vi "Cascade Logic.vi"(8 "Bank1 Status":T2, 9 "Bank1 Data":T4, 10 "Bank0 Status":T2, 11 "Bank0 Data":T4) -> (0 "Output Valid":bool, 3 "Output Data":T3, 4 "Cascaded Bank Status":T1)   [LabVIEW 2012]
doc: "This VI implements cascade logic to combine two DRAM Banks to act as a single FIFO.\nIt has the higher efficiency in throughput than Ping-Ponging between banks."
uses:
  <userlib>/FPGA Library/Code Development/DRAM/2 Bank DRAM/Data Type (256).ctl
  <userlib>/FPGA Library/Code Development/DRAM/2 Bank DRAM/Controls/Individual Bank Status.ctl
  <userlib>/FPGA Library/Code Development/DRAM/2 Bank DRAM/Controls/Cascaded Bank Status.ctl
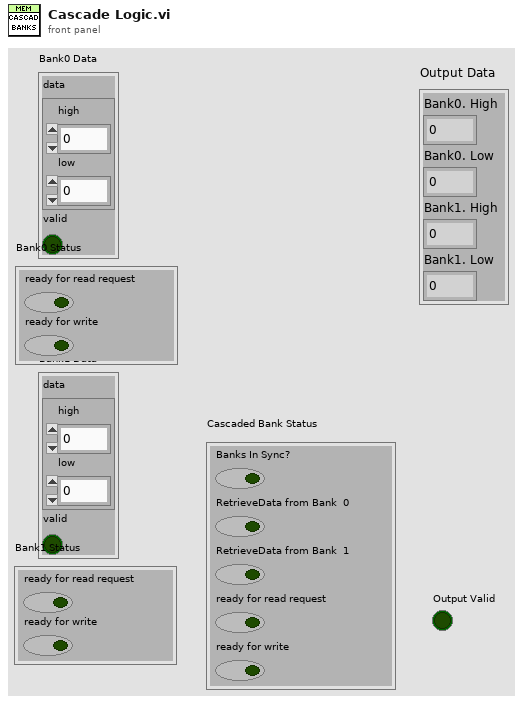
[diagram p1: front panel]
types:
  T1 = typedef "Cascaded Bank Status.ctl" = cluster{"Banks In Sync?":bool, "RetrieveData from Bank  0":bool, "RetrieveData from Bank  1":bool, "ready for read request":bool, "ready for write":bool}
  T2 = typedef "Individual Bank Status.ctl" = cluster{"ready for read request":bool, "ready for write":bool}
  T3 = typedef "Data Type (256).ctl" = cluster{"Bank0. High":u64, "Bank0. Low":u64, "Bank1. High":u64, "Bank1. Low":u64}
  T4 = cluster{"data":cluster{"high":u64, "low":u64}, "valid":bool}
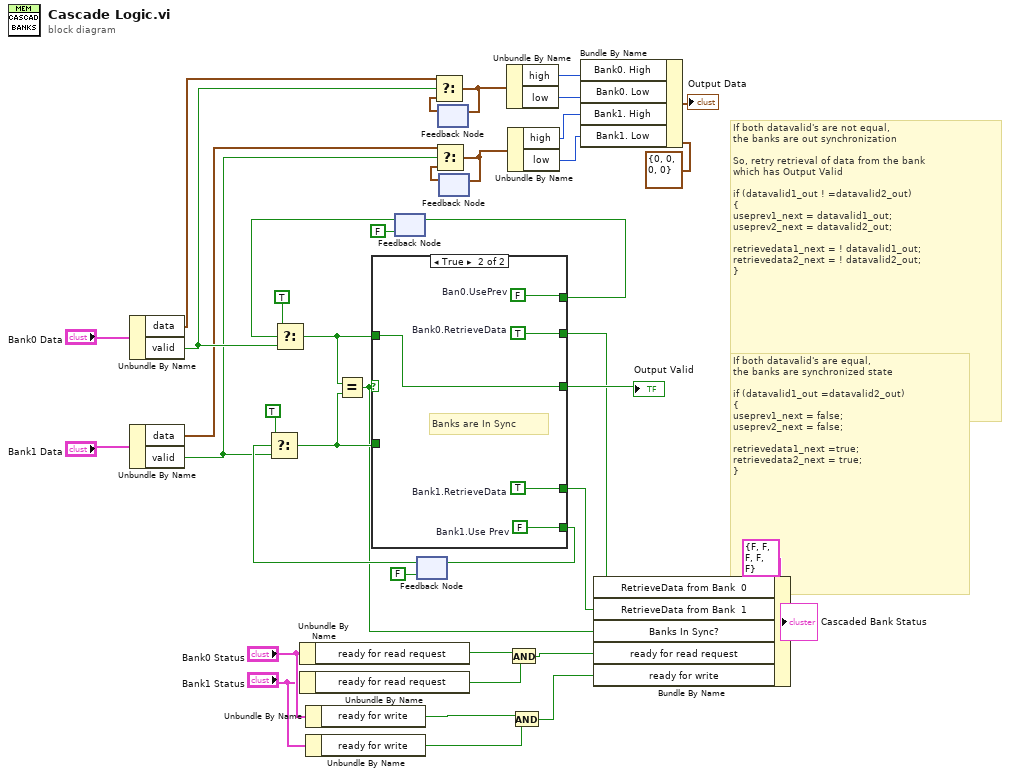
[diagram p0: block diagram]
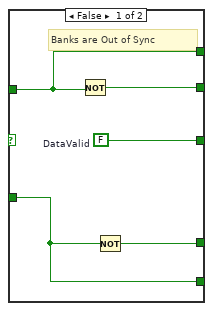
[diagram p2: hidden frame]
diagram:
  # "If both datavalid's are equal, \nthe banks are synchronized state\n\nif (datavalid1_out =datavalid2_out)\n{\nuseprev1_next = false;\nuseprev2_next = false;\n\nretrievedata1_next =true;\nretrievedata2_next = true;\n}"
  # "If both datavalid's are not equal, \nthe banks are out synchronization\n\nSo, retry retrieval of data from the bank \nwhich has Output Valid\n\nif (datavalid1_out ! =datavalid2_out)\n{\nuseprev1_next = datavalid1_out;\nuseprev2_next = datavalid2_out;\n\nretrievedata1_next = ! datavalid1_out;\nretrievedata2_next = ! datavalid2_out;\n}"
  n1 = Unbundle By Name("Bank0 Data") -> ("data"=w20:cluster{"high":u64, "low":u64}, "valid"=w21:bool)
  n2 = Unbundle By Name("Bank1 Data") -> ("data"=w14:cluster{"high":u64, "low":u64}, "valid"=w13:bool)
  n3 = Unbundle By Name("Bank0 Status") -> ("ready for read request"=w9:bool)
  n4 = Unbundle By Name("Bank1 Status") -> ("ready for read request"=w8:bool)
  n5 = Unbundle By Name("Bank0 Status") -> ("ready for write"=w4:bool)
  n6 = Unbundle By Name("Bank1 Status") -> ("ready for write"=w3:bool)
  n7 = feedback #1(FALSE ("Use Prev")) -> (w30:bool)
  n8 = Select(t=TRUE, s=w30, f=w21) -> (s? t:f=w39:bool)
  n9 = feedback #2(FALSE ("DataValid 2")) -> (w27:bool)
  n10 = Select(t=TRUE, s=w27, f=w13) -> (s? t:f=w37:bool)
  n11 = Equal?(x=w39, y=w37) -> (x = y?=w1:bool)
  n12 = case shown="True" w1 {
    tunnel: [w45 w50] -> w31
    tunnel: [w42 w47] -> w28
    tunnel: [w44 w48] -> w24
    tunnel: [w43 w49] -> w23
    tunnel: w39 -> [w45 w46]
    tunnel: w37 -> [w42 _]
    tunnel: [w41 w46] -> w34
    frame False {
      w41 = FALSE  # DataValid
      # "Banks are Out of Sync"
      n13 = Not(x=w45) -> (.not. x?=w44:bool)
      n14 = Not(x=w42) -> (.not. x?=w43:bool)
    }
    frame True {
      w47 = FALSE  # Bank1.Use Prev
      w48 = TRUE  # Bank0.RetrieveData
      w49 = TRUE  # Bank1.RetrieveData
      w50 = FALSE  # Ban0.UsePrev
      # "Banks are In Sync"
    }
  }
  "Output Valid" <- w34
  n15 = feedback-in #1(w31) -> ()
  n16 = feedback-in #2(w28) -> ()
  n17 = feedback #3() -> (w15:cluster{"high":u64, "low":u64})  [unwired: 1 in]
  n18 = Select(t=w20, s=w21, f=w15) -> (s? t:f=w19:cluster{"high":u64, "low":u64})
  n19 = feedback-in #3(w19) -> ()
  n20 = feedback #4() -> (w16:cluster{"high":u64, "low":u64})  [unwired: 1 in]
  n21 = Select(t=w14, s=w13, f=w16) -> (s? t:f=w12:cluster{"high":u64, "low":u64})
  n22 = feedback-in #4(w12) -> ()
  n23 = Unbundle By Name(w19) -> ("high"=w18:u64, "low"=w17:u64)
  n24 = Unbundle By Name(w12) -> ("high"=w11:u64, "low"=w10:u64)
  n25 = And(x=w9, y=w8) -> (x .and. y?=w7:bool)
  n26 = And(x=w4, y=w3) -> (x .and. y?=w2:bool)
  n27 = Bundle By Name(cluster=T3 {"Bank0. High"=0, "Bank0. Low"=0, "Bank1. High"=0, "Bank1. Low"=0} ("Output Data"), "Bank0. High"=w18, "Bank0. Low"=w17, "Bank1. High"=w11, "Bank1. Low"=w10) -> (→"Output Data":T3)
  n28 = Bundle By Name(cluster=T1 {"Banks In Sync?"=FALSE, "RetrieveData from Bank  0"=FALSE, "RetrieveData from Bank  1"=FALSE, "ready for read request"=FALSE, "ready for write"=FALSE} ("Cascaded Bank Status 2"), "RetrieveData from Bank  0"=w24, "RetrieveData from Bank  1"=w23, "Banks In Sync?"=w1, "ready for read request"=w7, "ready for write"=w2) -> (→"Cascaded Bank Status":T1)
